vi "Set Enable Debugging.vi"(8 "error in (no error)":errorcluster, 9 "Wait for debugger on launch (false)":bool, 10 "Enable debugging (false)":bool, 11 "EXE in":refnum<class "NI_AB_API_EXE.lvclass">) -> (0 "error out":errorcluster, 3 "EXE out":refnum<class "NI_AB_API_EXE.lvclass">)   [LabVIEW 2020, in "NI_AB_API_EXE.lvclass"]
uses:
  <vilib>/AppBuilder/AB_API/EXE/NI_AB_API_EXE.lvclass
  <vilib>/AppBuilder/AB_API/Application/NI_AB_API_Application.lvclass
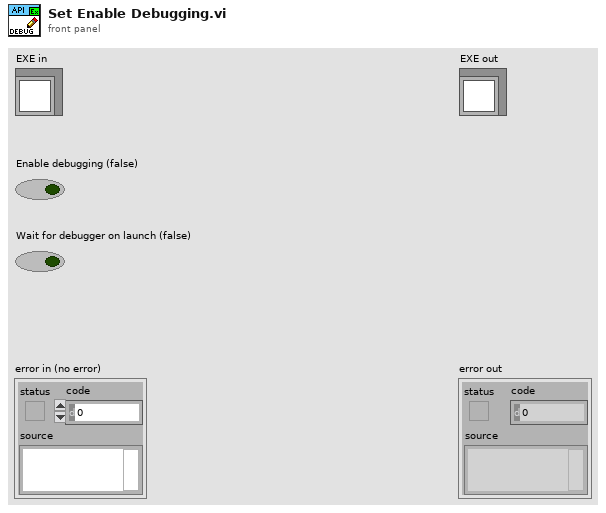
[diagram p1: front panel]
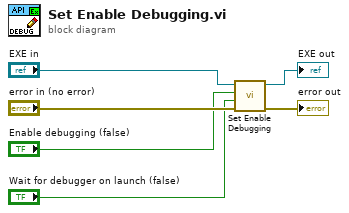
[diagram p0: block diagram]
diagram:
  n1 = call-parent "Set Enable Debugging.vi"("error in (no error)"="error in (no error)", "Wait for debugger on launch (false)"="Wait for debugger on launch (false)", "Enable debugging (false)"="Enable debugging (false)", "NI_AB_API_Application in"="EXE in") -> ("error out"=→"error out":errorcluster, "NI_AB_API_Application out"=→"EXE out":refnum<class "NI_AB_API_EXE.lvclass">)  [unwired: 6 in]
